vi "Read Resolution.vi"(8 "error in":errorcluster, 11 "Luminos in":refnum<class "Luminos.lvclass">) -> (0 "error out":errorcluster, 3 "Luminos out":refnum<class "Luminos.lvclass">)   [LabVIEW 2018, in "Luminos.lvlib" / "Luminos.lvclass"]
uses:
  Luminos.lvclass
  Luminos.lvclass/Luminos.ctl
  PPLs/Configuration/Configuration.lvlibp/Configuration.lvclass
  PPLs/Axis/Axis.lvlibp/Axis.lvclass
  C:/Projects/LabVIEW/PPLs/Axis/Axis.lvlibp/Axis.lvclass
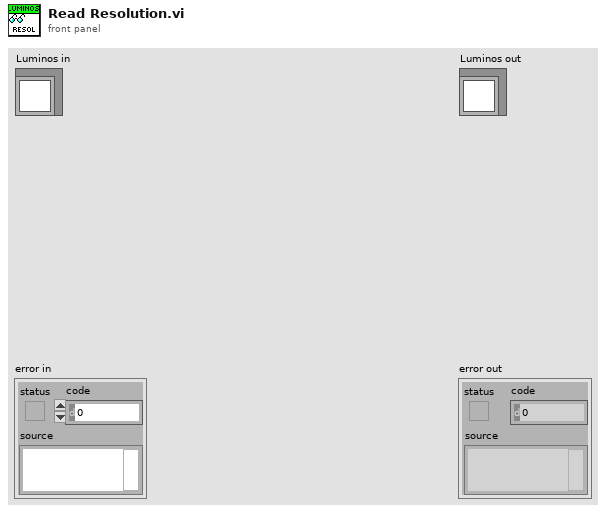
[diagram p1: front panel]
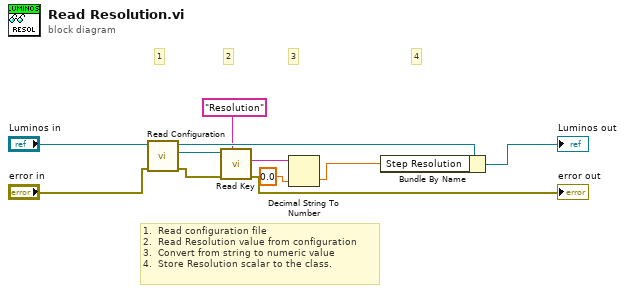
[diagram p0: block diagram]
diagram:
  # "1.  Read configuration file\n2.  Read Resolution value from configuration\n3.  Convert from string to numeric value\n4.  Store Resolution scalar to the class."
  # "4"
  # "3"
  # "2"
  # "1"
  n1 = call "Read Configuration.vi"("error in"="error in", "Axis in"="Luminos in") -> ("error out"=w6:errorcluster, "Configuration"=w10:refnum<class "Configuration.lvclass">, "Axis out"=w8:refnum<class "Luminos.lvclass">)  [unwired: 7 in]
  n2 = call "Read Key.vi"("Key:"="Resolution", "error in"=w6, "Configuration in"=w10) -> ("error out"=→"error out":errorcluster, "Value"=w9:string)  [unwired: 6 in, 1 out]
  n3 = Decimal String To Number(string=w9, default (0L)=0.0) -> (number=w2:dbl)  [unwired: 1 in, 1 out]
  n4 = Bundle By Name(cluster=w8, "Step Resolution"=w2) -> (→"Luminos out":refnum<class "Luminos.lvclass">)
